vi "save_timetrace_diag.vi"(9 "Boolean":bool, 10 "FilaPath":string, 11 "Numeric":dbl) -> (2 "path":path, 3 "Byte Stream File out":refnum<file>)   [LabVIEW 2013]
panel:
  out "string":string
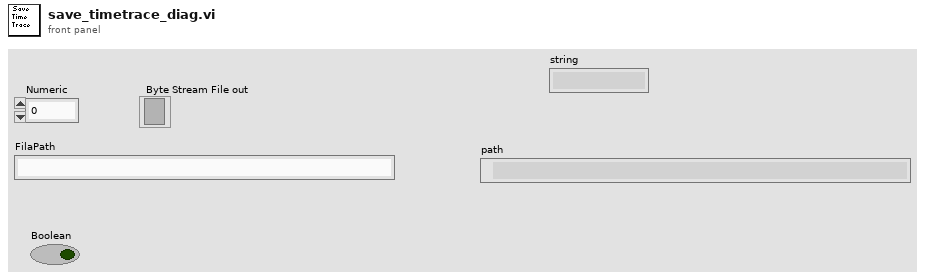
[diagram p1: front panel]
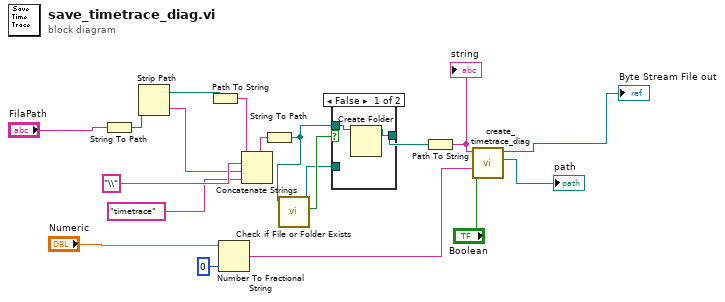
[diagram p0: block diagram]
diagram:
  n1 = String To Path(string="FilaPath") -> (path=w9:path)
  n2 = Strip Path(path=w9) -> (stripped path=w10:path, name=w3:string)
  n3 = Path To String(path=w10) -> (string=w11:string)
  n4 = Number To Fractional String(number="Numeric", precision (6)=i16 0) -> (F-format string=w7:string)  [unwired: 2 in]
  n5 = Concatenate Strings(w11, "\\" ("String"), w3, "timetrace" ("string")) -> (w17:string)
  n6 = String To Path(string=w17) -> (path=w13:path)
  n7 = call <vilib>:"Check if File or Folder Exists.vi"("path"=w13) -> ("file or folder exists?"=w15:bool, "dup path"=w14:path)  [unwired: 8 in, 1 out]
  n8 = case shown="False" w15 {
    tunnel: [w20 w22] -> w18
    tunnel: w14 -> [_ w22]
    tunnel: w13 -> [w21 _]
    frame False {
      n9 = Create Folder(path (use dialog)=w21) -> (created path=w20:path)  [unwired: 2 in, 2 out]
    }
    frame True {
    }
  }
  n10 = Path To String(path=w18) -> (string=w19:string)
  "string" <- w19
  n11 = call "create_timetrace_diag.vi"("Boolean"="Boolean", "string"=w7, "String"=w19) -> ("path"=→"path":path, "Byte Stream File out"=→"Byte Stream File out":refnum<file>)  [unwired: 7 in]
